vi "Build AI Table.vi"(11 "AI Node Ref In":i32) -> (1 "O PCT":dbl, 2 "X PCT":dbl, 3 "AI Node Ref Out":i32)   [LabVIEW 2013]
uses:
  Typedef/AI Table Node.ctl
  Typedef/Cell.ctl
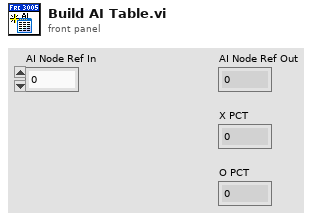
[diagram p1: front panel]
types:
  T1 = typedef "AI Table Node.ctl" = cluster{"Board State":i32, "Child Nodes":i32[], "X PCT":dbl, "O PCT":dbl, "Index":i32}
  T2 = typedef "Cell.ctl" = enum16{"", "X", "O"}
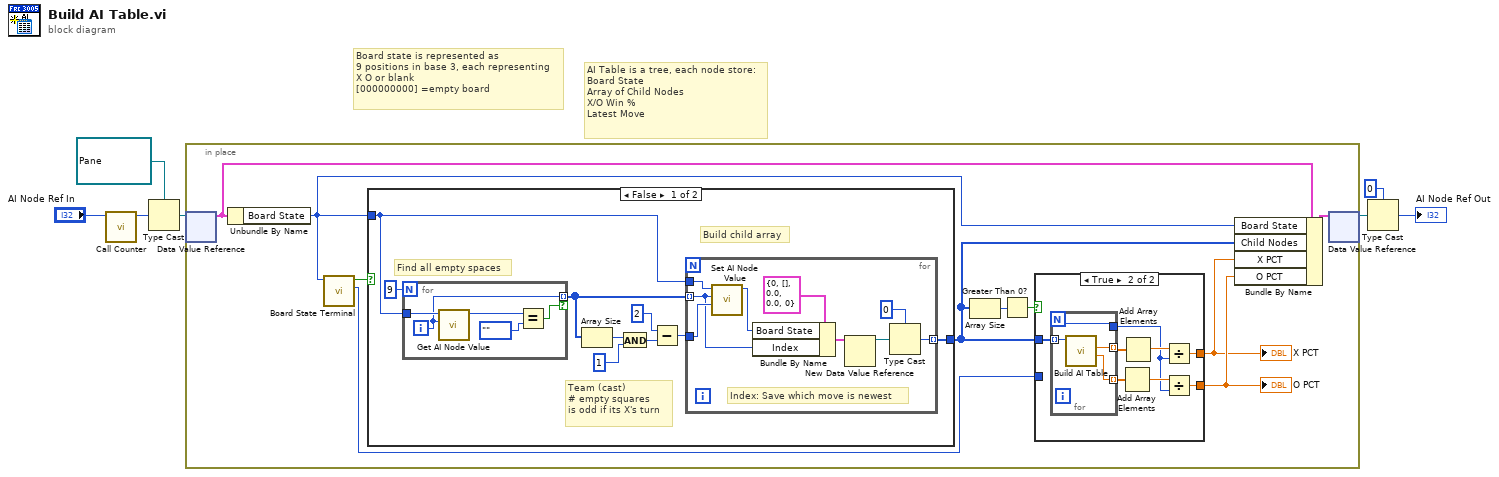
[diagram p0: block diagram]
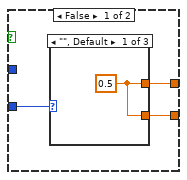
[diagram p2: hidden frame]
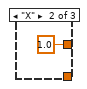
[diagram p3: hidden frame]
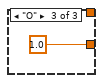
[diagram p4: hidden frame]
diagram:
  # "Board state is represented as\n9 positions in base 3, each representing\nX O or blank\n[000000000] =empty board"
  # "AI Table is a tree, each node store:\nBoard State\nArray of Child Nodes\nX/O Win %\nLatest Move"
  n1 = call "Call Counter.vi"("Ref In"="AI Node Ref In") -> ("Ref Out"=w1:i32)  [unwired: 9 in, 1 out]
  n2 = Type Cast(type=refnum<data-value> refnum ("data value reference"), x=w1) -> (*(type *) &x=w5:refnum<data-value>)
  n3 = in-place {
    n4 = in-place-dvr #1(w5) -> (w17:T1)  [unwired: 1 out]
    n5 = Unbundle By Name(w17) -> ("Board State"=w8:i32)
    n6 = call "Board State Terminal.vi"("Board State"=w8) -> ("Team"=w9:T2, "Terminal?"=w14:bool)  [unwired: 9 in]
    n7 = case shown="False" w14 {
      tunnel: w8 -> [w42 _]
      tunnel: [w41 _] -> w13
      frame False {
        # "Build child array"
        # "Team (cast)\n# empty squares\nis odd if its X's turn"
        # "Find all empty spaces"
        n8 = for {
          N: 9 -> [_]
          tunnel: w42 -> [w58]
          tunnel: [w54] -> w43 mode=indexing if=w55
          i -> [w54]
          n9 = call "Get AI Node Value.vi"("Location"=w54, "Board State"=w58) -> ("Value"=w56:T2)  [unwired: 9 in]
          n10 = Equal?(x=w56, y=Cell."" ("Value")) -> (x = y?=w55:bool)
        }
        n11 = Array Size(array=w43) -> (size(s)=w44:i32)
        n12 = And(x=w44, y=1) -> (x .and. y?=w38:i32)
        n13 = Subtract(x=2, y=w38) -> (x-y=w37:i32)
        n14 = for {
          tunnel: w43 -> [w45] mode=indexing
          tunnel: w37 -> [w52]
          tunnel: w42 -> [w51]
          tunnel: [w48] -> w41 mode=indexing
          # "Index: Save which move is newest"
          n15 = call "Set AI Node Value.vi"("Value"=w52, "Location"=w45, "Board State In"=w51) -> ("Board State Out"=w46:i32)  [unwired: 8 in]
          n16 = Bundle By Name(cluster=T1 {"Board State"=0, "Child Nodes"=[], "X PCT"=0.0, "O PCT"=0.0, "Index"=0} ("data value"), "Board State"=w46, "Index"=w45) -> (w50:T1)
          n17 = New Data Value Reference(data value=w50) -> (data value reference=w49:refnum<data-value>)  [unwired: 1 in, 1 out]
          n18 = Type Cast(type=0 ("y"), x=w49) -> (*(type *) &x=w48:i32)
        }
      }
      frame True {
        # "Dont recurse if this is a terminal board"
      }
    }
    n19 = Array Size(array=w13) -> (size(s)=w15:i32)
    n20 = Greater Than 0?(x=w15) -> (x > 0?=w12:bool)
    n21 = case shown="True" w12 {
      tunnel: w13 -> [_ w31]
      tunnel: [w18 w25] -> w10
      tunnel: [w19 w24] -> w11
      tunnel: w9 -> [w20 _]
      frame False {
        n22 = case shown="\"\", Default" w20 {
          tunnel: [w21 _ 1.0] -> w19
          tunnel: [w21 1.0 _] -> w18
          frame "", Default {
            w21 = 0.5
          }
          frame "X" {
          }
          frame "O" {
          }
        }
      }
      frame True {
        n23 = for {
          N -> [w32]
          tunnel: w31 -> [w35] mode=indexing
          tunnel: [w34] -> w29 mode=indexing
          tunnel: [w33] -> w30 mode=indexing
          tunnel: [w32] -> w26
          n24 = call "Build AI Table.vi"("AI Node Ref In"=w35) -> ("O PCT"=w34:dbl, "X PCT"=w33:dbl)  [unwired: 8 in, 1 out]
        }
        n25 = Add Array Elements(numeric array=w29) -> (sum=w27:dbl)
        n26 = Add Array Elements(numeric array=w30) -> (sum=w28:dbl)
        n27 = Divide(x=w28, y=w26) -> (x/y=w25:dbl)
        n28 = Divide(x=w27, y=w26) -> (x/y=w24:dbl)
      }
    }
    "O PCT" <- w11
    "X PCT" <- w10
    n29 = Bundle By Name(cluster=w17, "Board State"=w8, "Child Nodes"=w13, "X PCT"=w10, "O PCT"=w11) -> (w16:T1)
    n30 = in-place-dvr #1(w16) -> (w7:refnum<data-value>)  [unwired: 1 out]
  }
  n31 = Type Cast(type=0 ("y"), x=w7) -> (*(type *) &x=→"AI Node Ref Out":i32)
